vi "c_ctre_phoenix6_platform_start_logger.vi"() -> (20 "Numeric":i32)   [LabVIEW 2023]
uses:
  <vilib>/Rock Robotics/WPI/ThirdParty/Phoenix-LabVIEW/Controls/DriverLib.ctl
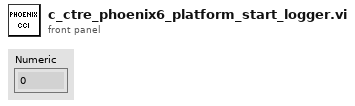
[diagram p1: front panel]
types:
  T1 = typedef "DriverLib.ctl" = path
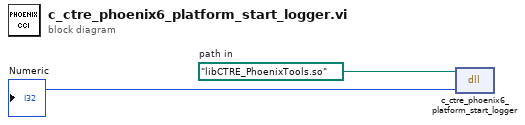
[diagram p0: block diagram]
diagram:
  w2 = T1 path "libCTRE_PhoenixTools.so"  # path in
  n1 = dll-call lib="?" fn="c_ctre_phoenix6_platform_start_logger"(path in=w2) -> (→"Numeric":i32)  [unwired: 2 in, 2 out]
